vi "Record2DAQ.vi"(0 "instrument in":T2, 1 "Additional text":string, 2 "numSamples":i32=-1, 5 "File location":path, 7 "Type of\nmeasurement":T3, 9 "Name root":string, 11 "error in":errorcluster, 12 "Run":string, 14 "number of files":i32) -> (3 "output cluster":T1, 4 "instrument out":T2, 6 "waveform":waveform(dbl)[](array[waveform]), 10 "File count":i32, 15 "error out":errorcluster)   [LabVIEW 2013]
uses:
  Strict Type Defs/type_meas_enum.ctl
  <instrlib>/niScope/Acquire/Fetch/niScope Fetch Binary 16.vi
  <instrlib>/niScope/Acquire/Fetch/niScope Multi Fetch Binary 16.vi
panel:
  out "Chan 2 params":T4
  out "Chan 1 params":T4
  out "Chan 0 params":T4
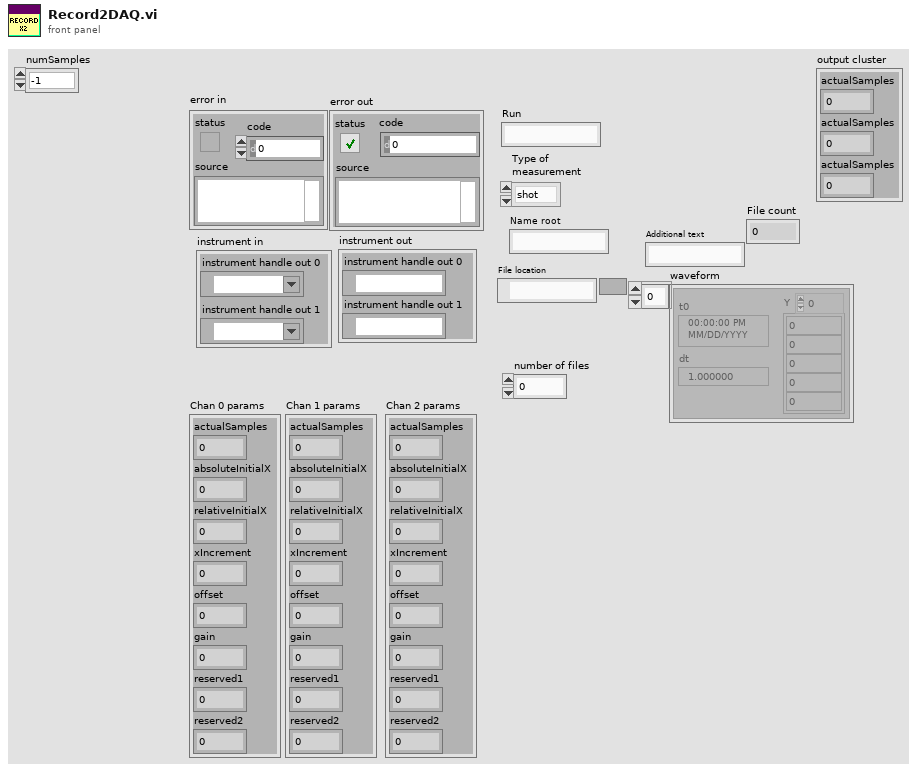
[diagram p1: front panel]
types:
  T1 = cluster{"actualSamples":i32, "actualSamples":i32, "actualSamples":i32}
  T2 = cluster{"instrument handle out 0":refnum<k15>, "instrument handle out 1":refnum<k15>}
  T3 = typedef "type_meas_enum.ctl" = enum16{"shot", "x", "p", "electronic"}
  T4 = cluster{"actualSamples":i32, "absoluteInitialX":dbl, "relativeInitialX":dbl, "xIncrement":dbl, "offset":dbl, "gain":dbl, "reserved1":dbl, "reserved2":dbl}
  T5 = cluster{"actualSamples":i32, "absoluteInitialX":dbl, "relativeInitialX":dbl, "xIncrement":dbl, "offset":dbl, "gain":dbl, "reserved1":dbl, "reserved2":dbl}[]
  T6 = cluster{"instrument handle out":refnum<k15>, "instrument handle out":refnum<k15>}
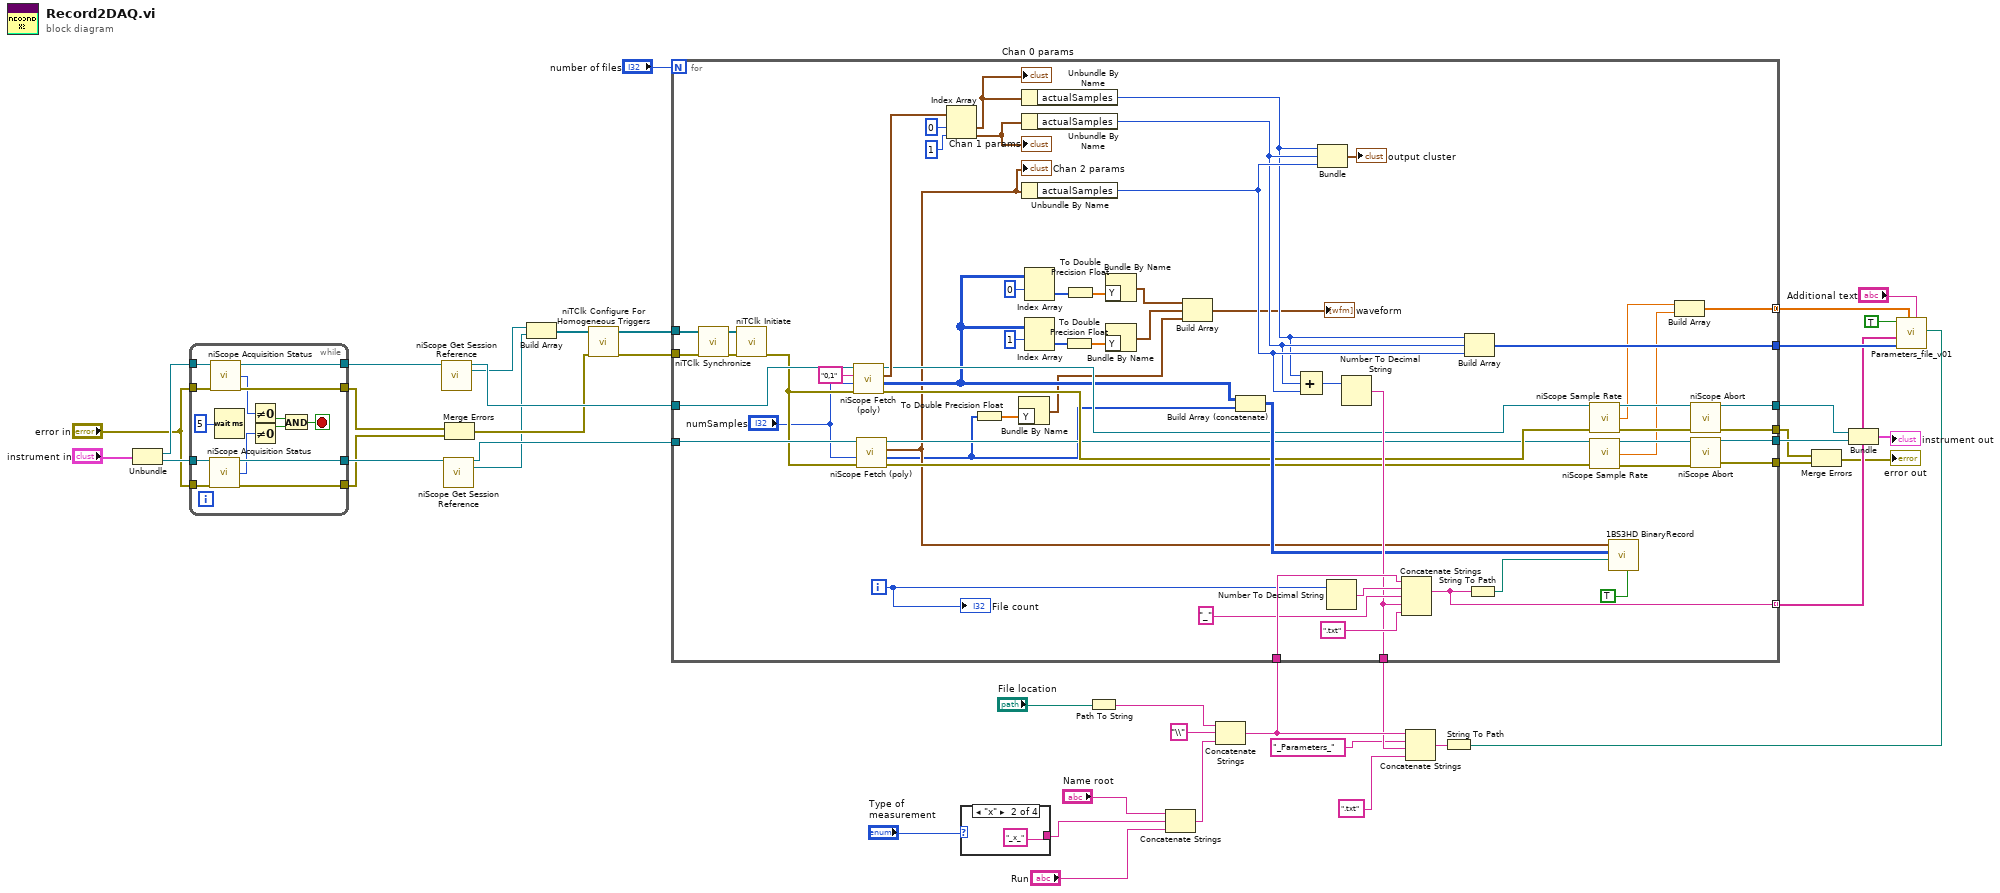
[diagram p0: block diagram]
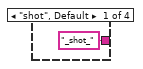
[diagram p2: hidden frame]
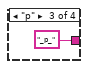
[diagram p3: hidden frame]
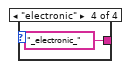
[diagram p4: hidden frame]
diagram:
  n1 = Unbundle("instrument in") -> ("instrument handle out 0"=w22:refnum<k15>, "instrument handle out 1"=w21:refnum<k15>)
  n2 = while {
    tunnel: w22 -> [w55]
    tunnel: "error in" -> [w54]
    tunnel: w21 -> [w52]
    tunnel: "error in" -> [w49]
    tunnel: [w56] -> w4
    tunnel: [w53] -> w3
    tunnel: [w51] -> w2
    tunnel: [w50] -> w1
    stop <- w44 stop-if-true
    n3 = call <instrlib>:"niScope Acquisition Status.vi"("instrument handle"=w52, "error in"=w49) -> ("instrument handle out"=w51:refnum<k15>, "acquisition status"=w48:i32, "error out"=w50:errorcluster)  [unwired: 11 in]
    n4 = call <instrlib>:"niScope Acquisition Status.vi"("instrument handle"=w55, "error in"=w54) -> ("instrument handle out"=w56:refnum<k15>, "acquisition status"=w47:i32, "error out"=w53:errorcluster)  [unwired: 11 in]
    n5 = Wait (ms)(milliseconds to wait=u32 5) -> ()  [unwired: 1 out]
    n6 = Not Equal To 0?(x=w47) -> (x != 0?=w46:bool)
    n7 = Not Equal To 0?(x=w48) -> (x != 0?=w45:bool)
    n8 = And(x=w46, y=w45) -> (x .and. y?=w44:bool)
  }
  n9 = call <instrlib>:"niScope Get Session Reference.vi"("instrument handle"=w4) -> ("instrument handle out"=w16:refnum<k15>, "session reference"=w5:refnum<k20>)  [unwired: 12 in, 1 out]
  n10 = call <instrlib>:"niScope Get Session Reference.vi"("instrument handle"=w2) -> ("instrument handle out"=w15:refnum<k15>, "session reference"=w10:refnum<k20>)  [unwired: 12 in, 1 out]
  n11 = Merge Errors(w3, w1) -> (w12:errorcluster)
  n12 = Build Array(w5, w10) -> (w11:refnum<k20>[])
  n13 = call <instrlib>:"niTClk Configure For Homogeneous Triggers.vi"("error in (no error)"=w12, "sessions"=w11) -> ("error out"=w13:errorcluster, "sessions out"=w14:refnum<k20>[])  [unwired: 8 in]
  n14 = case shown="\"x\"" "Type of\nmeasurement" {
    tunnel: ["_shot_" "_x_" "_p_" "_electronic_"] -> w32
    frame "shot", Default {
    }
    frame "x" {
    }
    frame "p" {
    }
    frame "electronic" {
    }
  }
  n15 = Path To String(path="File location") -> (string=w36:string)
  n16 = Concatenate Strings("Name root", w32, "Run") -> (w33:string)
  n17 = Concatenate Strings(w36, "\\" ("string"), w33) -> (w29:string)
  n18 = for {
    N: "number of files" -> [_]
    tunnel: [w109] -> w39
    tunnel: w29 -> [w110]
    tunnel: [w106] -> w30 mode=indexing
    tunnel: [w103] -> w26
    tunnel: w16 -> [w94]
    tunnel: [w102] -> w19
    tunnel: w15 -> [w97]
    tunnel: [w101] -> w18
    tunnel: [w100] -> w8
    tunnel: [w98] -> w7
    tunnel: w14 -> [w92]
    tunnel: w13 -> [w91]
    tunnel: [w80] -> w6 mode=concatenating
    i -> [w61]
    n19 = call <instrlib>:"niTClk Synchronize.vi"("error in (no error)"=w91, "sessions"=w92) -> ("error out"=w96:errorcluster, "sessions out"=w95:refnum<k20>[])  [unwired: 8 in]
    n20 = call <instrlib>:"niTClk Initiate.vi"("error in (no error)"=w96, "sessions"=w95) -> ("error out"=w93:errorcluster)  [unwired: 8 in, 1 out]
    n21 = call-poly <instrlib>:"niScope Fetch (poly).vi"("error in"=w93, "numSamples"="numSamples", "channels"="0,1", "instrument handle"=w94) -> ("error out"=w89:errorcluster, "wfm"=w75:i16[][], "wfm info"=w112:T5, "instrument handle out"=w90:refnum<k15>)  [unwired: 1 in, 3 out]
    n22 = call-poly <instrlib>:"niScope Fetch (poly).vi"("error in"=w93, "numSamples"="numSamples", "instrument handle"=w97) -> ("error out"=w84:errorcluster, "wfm"=w69:i16[], "wfm info"=w70:T4, "instrument handle out"=w85:refnum<k15>)  [unwired: 2 in, 3 out]
    "Chan 2 params" <- w70
    n23 = Index Array(array=w112, index #1=0 ("index"), index #2=1 ("index")) -> (element #1=w114:T4, element #2=w113:T4)
    "Chan 0 params" <- w114
    "Chan 1 params" <- w113
    n24 = To Double Precision Float(number=w69) -> (double precision float=w68:dbl[])
    n25 = Bundle By Name("Y"=w68) -> (w65:waveform(dbl))  [unwired: 1 in]
    n26 = Unbundle By Name(w114) -> ("actualSamples"=w77:i32)
    n27 = Unbundle By Name(w113) -> ("actualSamples"=w78:i32)
    n28 = Unbundle By Name(w70) -> ("actualSamples"=w79:i32)
    n29 = Index Array(array=w75, index (row)=0 ("index")) -> (element=w74:i16[])  [unwired: 1 in]
    n30 = Index Array(array=w75, index (row)=1 ("index")) -> (element=w72:i16[])  [unwired: 1 in]
    n31 = To Double Precision Float(number=w72) -> (double precision float=w71:dbl[])
    n32 = To Double Precision Float(number=w74) -> (double precision float=w73:dbl[])
    n33 = Bundle By Name("Y"=w73) -> (w67:waveform(dbl))  [unwired: 1 in]
    n34 = Bundle By Name("Y"=w71) -> (w66:waveform(dbl))  [unwired: 1 in]
    n35 = Build Array(w67, w66, w65) -> (→"waveform":waveform(dbl)[])
    n36 = Build Array (concatenate)(w75, w69) -> (w99:i16[][])
    n37 = Compound Arithmetic op=ADD(w77, w78, w79) -> (w108:i32)
    n38 = Bundle("actualSamples"=w77, "actualSamples"=w78, "actualSamples"=w79) -> (→"output cluster":T1)  [unwired: 1 in]
    n39 = Number To Decimal String(number=w61) -> (decimal integer string=w111:string)  [unwired: 1 in]
    n40 = Number To Decimal String(number=w108) -> (decimal integer string=w103:string)  [unwired: 1 in]
    n41 = Concatenate Strings(w110, w111, "_" ("string"), w103, ".txt") -> (w106:string)
    n42 = Build Array(w77, w78, w79) -> (w109:i32[])
    n43 = String To Path(string=w106) -> (path=w107:path)
    n44 = call <instrlib>:"niScope Sample Rate.vi"("instrument handle"=w90, "error in"=w89) -> ("instrument handle out"=w87:refnum<k15>, "actual sample rate"=w82:dbl, "error out"=w88:errorcluster)  [unwired: 11 out]
    n45 = call <instrlib>:"niScope Sample Rate.vi"("instrument handle"=w85, "error in"=w84) -> ("instrument handle out"=w86:refnum<k15>, "actual sample rate"=w81:dbl, "error out"=w83:errorcluster)  [unwired: 11 out]
    n46 = call "1BS3HD BinaryRecord.vi"("Record"=TRUE, "File name"=w107, "wfm"=w99, "Chan params"=w70) -> ()  [unwired: 8 in]
    n47 = Build Array(w82, w81) -> (w80:dbl[])
    n48 = call <instrlib>:"niScope Abort.vi"("instrument handle"=w87, "error in"=w88) -> ("instrument handle out"=w102:refnum<k15>, "error out"=w100:errorcluster)  [unwired: 12 in]
    n49 = call <instrlib>:"niScope Abort.vi"("instrument handle"=w86, "error in"=w83) -> ("instrument handle out"=w101:refnum<k15>, "error out"=w98:errorcluster)  [unwired: 12 in]
    "File count" <- w61
  }
  n50 = Concatenate Strings(w29, "_Parameters_" ("string"), w26, ".txt") -> (w28:string)
  n51 = String To Path(string=w28) -> (path=w27:path)
  n52 = Merge Errors(w8, w7) -> (→"error out":errorcluster)
  n53 = Bundle("instrument handle out"=w19, "instrument handle out"=w18) -> (→"instrument out":T6)  [unwired: 1 in]
  n54 = call "Parameters_file_v01.vi"("Additional text"="Additional text", "actual sample rate array"=w6, "actualSamples array"=w39, "Files name array"=w30, "File location"=w27, "Record"=TRUE) -> ()  [unwired: 3 in, 1 out]
